vi "Program_Active.vi"(0 "Hit Server Now":bool) -> ()   [LabVIEW 2010]
uses:
  ADAM Controls/Traverse_Level_State.ctl
  Anemometry/Anemometry Sub Vis/Globals/Meas_global.vi
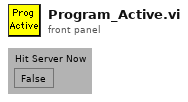
[diagram p1: front panel]
types:
  T1 = typedef "Post_Process.ctl" = enum16{"Take New Data", "Post Process Raw Data File"}
  T2 = typedef "Traverse_Level_State.ctl" = enum16{"Running", "Complete"}
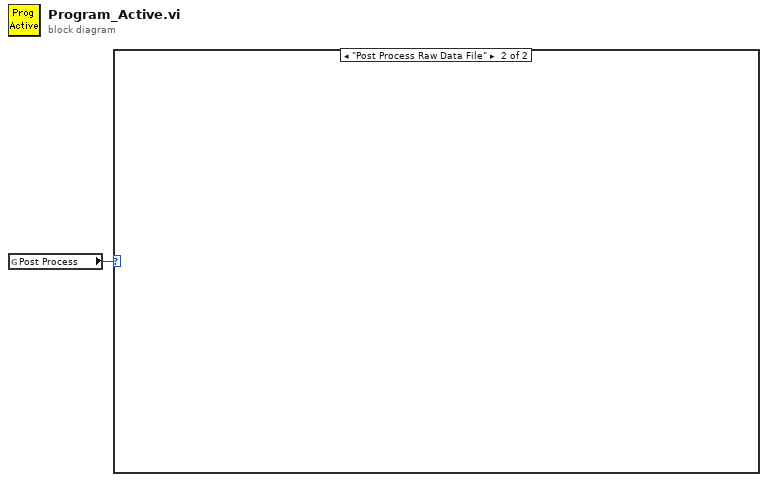
[diagram p0: block diagram]
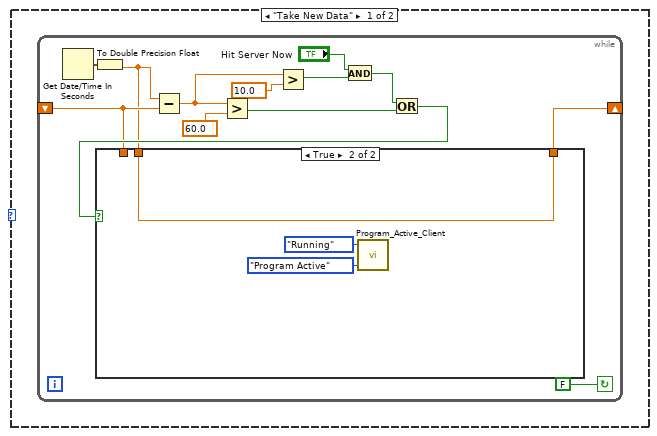
[diagram p2: hidden frame]
diagram:
  n1 = global read "Meas_global.vi" "Post Process"() -> (w1:T1)
  n2 = case shown="\"Post Process Raw Data File\"" w1 {
    frame "Take New Data" {
      n3 = while {
        shift-left: _ -> [w10]
        shift-right: [w11] -> _
        stop <- FALSE continue-if-true
        n4 = Get Date/Time In Seconds() -> (seconds since 1Jan1904=w2:timestamp)
        n5 = To Double Precision Float(number=w2) -> (double precision float=w9:dbl)
        n6 = Subtract(x=w9, y=w10) -> (x-y=w8:dbl)
        n7 = Greater?(x=w8, y=60.0) -> (0:w13:bool)
        n8 = Greater?(x=w8, y=10.0) -> (0:w5:bool)
        n9 = And(x="Hit Server Now", y=w5) -> (x .and. y?=w4:bool)
        n10 = Or(x=w4, y=w13) -> (x .or. y?=w12:bool)
        n11 = case shown="True" w12 {
          tunnel: [w15 w17] -> w11
          tunnel: w9 -> [_ w17]
          tunnel: w10 -> [w15 _]
          frame False {
          }
          frame True {
            n12 = call "Program_Active_Client.vi"("Mode"=enum16{"Program Active", "Traverse Level State"}."Program Active", "Traverse level State"=Traverse_Level_State."Running") -> ()  [unwired: 1 in, 3 out]
          }
        }
      }
    }
    frame "Post Process Raw Data File" {
    }
  }
